vi "PH_Cam_BaseClass.get Image Position Path.vi"(1 "i ref in":refnum<vi>) -> (0 "Image GUI Postion Path":path)   [LabVIEW 2014, in "PH_Cam_BaseClass.lvlib"]
doc: "This VI sets the path to get or to set the position of the GUI image to a xml-file."
uses:
  PH_Cam_BaseClass.lvlib
  PH_Common/PH_Common.lvlib
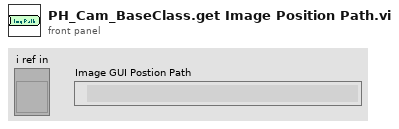
[diagram p1: front panel]
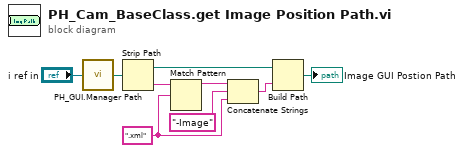
[diagram p0: block diagram]
diagram:
  w2 = ".xml" ("regular expression")
  n1 = call "PH_GUI.Manager Path.vi"("i ref in"="i ref in") -> ("GUI Manager Path"=w9:path)
  n2 = Strip Path(path=w9) -> (stripped path=w5:path, name=w8:string)
  n3 = Match Pattern(string=w8, regular expression=w2) -> (before substring=w7:string)  [unwired: 1 in, 3 out]
  n4 = Concatenate Strings(w7, "-Image" ("string"), w2) -> (w4:string)
  n5 = Build Path(base path=w5, name or relative path=w4) -> (appended path=→"Image GUI Postion Path":path)
